vi "Queue Flush.vi"(8 "error in (no error)":errorcluster, 11 "queue name in":string) -> (0 "error out":errorcluster)   [LabVIEW 2020]
uses:
  Control/Queue Data.ctl
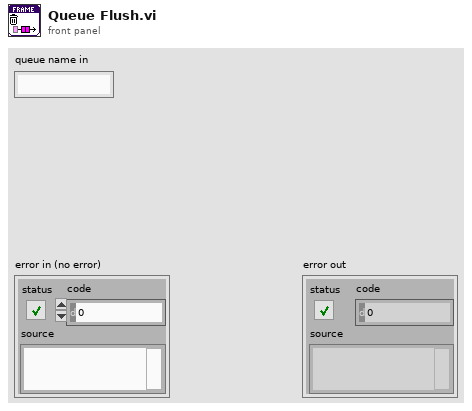
[diagram p1: front panel]
types:
  T1 = typedef "Queue Data.ctl" = cluster{"event":string, "data":variant}
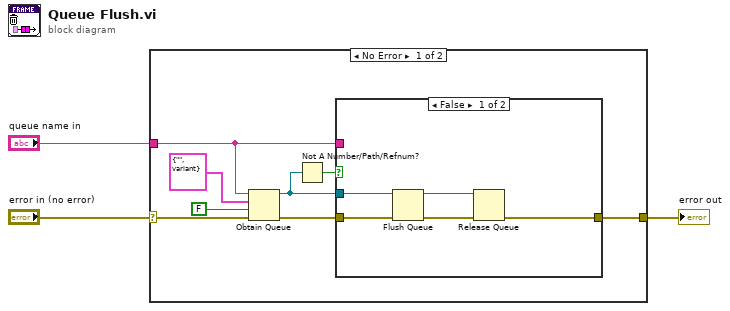
[diagram p0: block diagram]
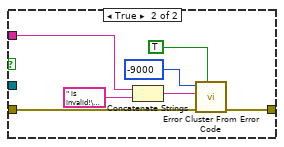
[diagram p2: hidden frame]
diagram:
  n1 = case shown="No Error" "error in (no error)" {
    selector: "error in (no error)" -> [w11 w24]
    tunnel: [w4 w24] -> w2
    tunnel: "queue name in" -> [w5 _]
    frame No Error {
      n2 = Obtain Queue(name (unnamed)=w5, element data type=T1 {"event"="", "data"=variant}, create if not found? (T)=FALSE, error in (no error)=w11) -> (queue out=w7:refnum<queue>, error out=w8:errorcluster)  [unwired: 1 in, 1 out]
      n3 = Not A Number/Path/Refnum?(number/path/refnum=w7) -> (NaN/Path/Refnum?=w6:bool)
      n4 = case shown="False" w6 {
        tunnel: w8 -> [w16 w19]
        tunnel: w7 -> [w15 _]
        tunnel: w5 -> [_ w18]
        tunnel: [w12 w17] -> w4
        frame False {
          n5 = Flush Queue(queue=w15, error in (no error)=w16) -> (queue out=w13:refnum<queue>, error out=w14:errorcluster)  [unwired: 1 out]
          n6 = Release Queue(queue=w13, error in (no error)=w14) -> (error out=w12:errorcluster)  [unwired: 1 in, 2 out]
        }
        frame True {
          n7 = Concatenate Strings(w18, " is invalid!\nEnsure the queue has been created!" ("字符串")) -> (w23:string)
          n8 = call <vilib>:"Error Cluster From Error Code.vi"("show call chain? (False)"=TRUE, "error in (no error)"=w19, "error message (\"\")"=w23, "error code (0)"=-9000) -> ("error out"=w17:errorcluster)  [unwired: 5 in]
        }
      }
    }
    frame Error {
    }
  }
  "error out" <- w2
